vi "THDReport.vi"(8 "error in (no error)":errorcluster, 11 "THD+N Array":string[][](array[string])) -> (0 "error out":errorcluster)   [LabVIEW 2014]
uses:
  typedefs/ePathsAction.ctl
  Excel(ActiveX)/enumOpenOrCreate.ctl
  Excel(ActiveX)/Excel(ActiveX).lvlib
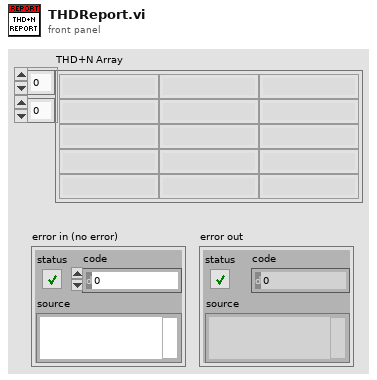
[diagram p1: front panel]
types:
  T1 = typedef "Excel(ActiveX).lvlib/enumOpenOrCreate.ctl" = enum16{"open", "open or create", "create from template"}
  T2 = typedef "ePathsAction.ctl" = enum16{"Set", "Get", "Load", "Save", "Default", "Exit"}
  T3 = typedef "Paths.ctl" = cluster{"BasePath":path, "FlukePath":path, "LastFlukePath":path, "NISTPath":path, "LastNISTPath":path, "ResultsPath":path}
  T4 = typedef "Excel(ActiveX).lvlib/ExcelActiveX.ctl" = cluster{"Excel._Application":refnum<k7>, "Application open at start":bool, "Excel._Worksheet":refnum<k7>, "Workbook open at start":bool, "Excel._Workbook":refnum<k7>, "Workbook Path":path, "Worksheet Name":string, "Row":u32, "Col":u32, "Cell":string, "Workbook Name":string}
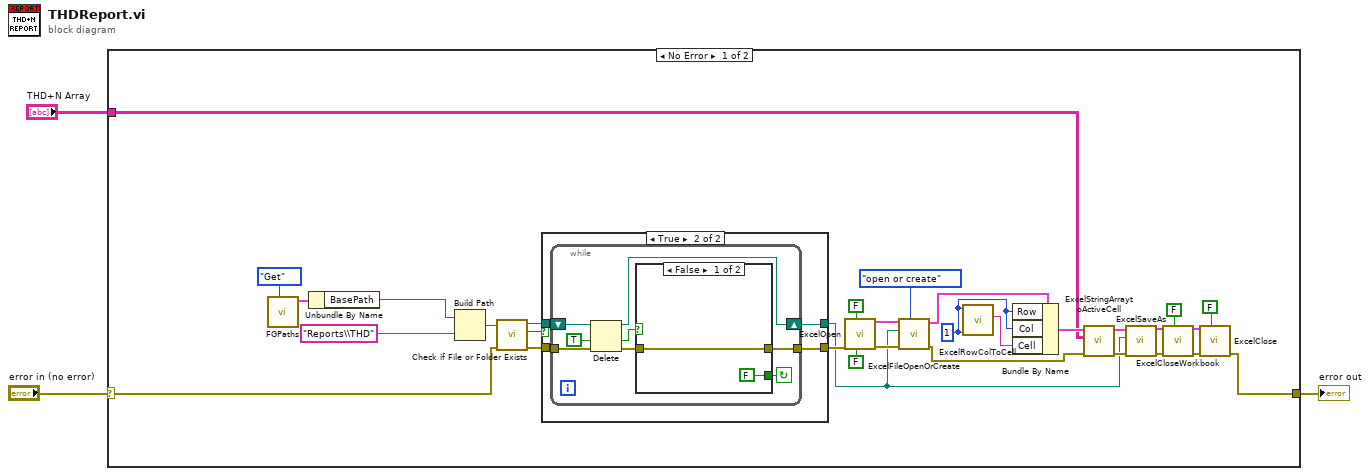
[diagram p0: block diagram]
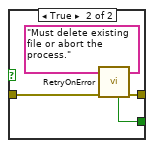
[diagram p3: hidden frame]
diagram:
  n1 = case shown="No Error" "error in (no error)" {
    selector: "error in (no error)" -> [w5 w55]
    tunnel: [w8 w55] -> w2
    tunnel: "THD+N Array" -> [w4 _]
    frame No Error {
      w19 = u32 1 ("col")
      n2 = call "FGPaths.vi"("ePathsAction"=ePathsAction."Get") -> ("PathsOut"=w33:T3)  [unwired: 9 in, 1 out]
      n3 = Unbundle By Name(w33) -> ("BasePath"=w32:path)
      n4 = Build Path(base path=w32, name or relative path="Reports\\THD" ("message")) -> (appended path=w28:path)
      n5 = call <vilib>:"Check if File or Folder Exists.vi"("error in (no error)"=w5, "path"=w28) -> ("error out"=w29:errorcluster, "file or folder exists?"=w31:bool, "dup path"=w30:path)  [unwired: 7 in]
      n6 = case shown="True" w31 {
        tunnel: w30 -> [w35 w40]
        tunnel: w29 -> [w36 w39]
        tunnel: [w36 w37] -> w23
        tunnel: [w35 w38] -> w7
        frame False {
        }
        frame True {
          n7 = while {
            shift-right: [w45] -> w38
            shift-left: w40 -> [w47]
            tunnel: w39 -> [w46]
            tunnel: [w43] -> w37
            stop <- w41 continue-if-true
            n8 = Delete(path (use dialog)=w47, confirm (F)=TRUE, error in=w46) -> (deleted path=w45:path, cancelled=w42:bool, error out=w44:errorcluster)  [unwired: 2 in]
            n9 = case shown="False" w42 {
              tunnel: w44 -> [w50 w52]
              tunnel: [w50 w54] -> w43
              tunnel: [FALSE ("Retry") w53] -> w41
              frame False {
              }
              frame True {
                n10 = call "RetryOnError.vi"("error in (no error)"=w52, "Error Msg"="Must delete existing file or abort the process.") -> ("error out"=w54:errorcluster, "Retry"=w53:bool)  [unwired: 8 in]
              }
            }
          }
        }
      }
      n11 = call "ExcelOpen.vi"("Run Minimized (f)"=FALSE, "Excel visible? (t)"=FALSE, "error in (no error)"=w23) -> ("error out"=w26:errorcluster, "ExcelActiveX"=w27:T4)  [unwired: 7 in]
      n12 = call "ExcelFileOpenOrCreate.vi"("Open or Create"=enumOpenOrCreate."open or create", "error in (no error)"=w26, "Excel file name and path"=w7, "ExcelActiveX in"=w27) -> ("error out"=w18:errorcluster, "ExcelActiveX out"=w21:T4)  [unwired: 6 in]
      n13 = call "ExcelRowColToCell.vi"("col"=w19, "row"=w19) -> ("cell"=w20:string)  [unwired: 9 in]
      n14 = Bundle By Name(cluster=w21, "Row"=w19, "Col"=w19, "Cell"=w20) -> (w17:T4)
      n15 = call "ExcelStringArraytoActiveCell.vi"("error in (no error)"=w18, "Array"=w4, "ExcelActiveX"=w17) -> ("error out"=w10:errorcluster, "ExcelActiveX"=w9:T4)  [unwired: 7 in]
      n16 = call "ExcelSaveAs.vi"("error in (no error)"=w10, "Path"=w7, "ExcelActiveX"=w9) -> ("error out"=w15:errorcluster, "ExcelActiveX"=w13:T4)  [unwired: 7 in]
      n17 = call "ExcelCloseWorkbook.vi"("Save"=FALSE, "error in (no error)"=w15, "ExcelActiveX"=w13) -> ("error out"=w14:errorcluster, "ExcelActiveX"=w12:T4)  [unwired: 7 in]
      n18 = call "ExcelClose.vi"("Leave Open (f)"=FALSE, "error in (no error)"=w14, "ExcelActiveX in"=w12) -> ("error out"=w8:errorcluster)  [unwired: 7 in, 1 out]
    }
    frame Error {
    }
  }
  "error out" <- w2
